vi "Anritsu VNA Read Trigger Mode.vi"(6 "Channel":i8=1 min=1 max=99 step=1, 7 "Anritsu VNA":T1, 8 "error in (no error)":errorcluster, 11 "VISA Resource Name":refnum<visa-resource-name>) -> (0 "error out":errorcluster, 2 "Trigger Mode":T2, 3 "dup VISA Resource Name":refnum<visa-resource-name>)   [LabVIEW 2011]
doc: "This VI for the HP8753B Network Analyzers reads the stimulus values. Except when performing log sweeps and freq list sweeps, this VI uses the start and stop values and the number of points to calcuate the stimulus values."
uses:
  TypeDefs/Anritsu VNA Trigger Mode.ctl
  TypeDefs/Anritsu VNA Instrument Info.ctl
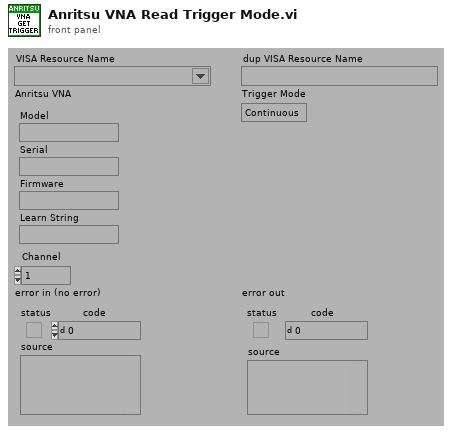
[diagram p1: front panel]
types:
  T1 = typedef "Anritsu VNA Instrument Info.ctl" = cluster{"Model":string, "Serial":string, "Firmware":string, "Learn String":string}
  T2 = typedef "Anritsu VNA Trigger Mode.ctl" = enum16{"Continuous", "Hold", "Single"}
  T3 = typedef "Anritsu VNA Model.ctl" = enum16{"Not Supported", "37XXXX", "MS20XXX", "MS462XX", "MS464XX"}
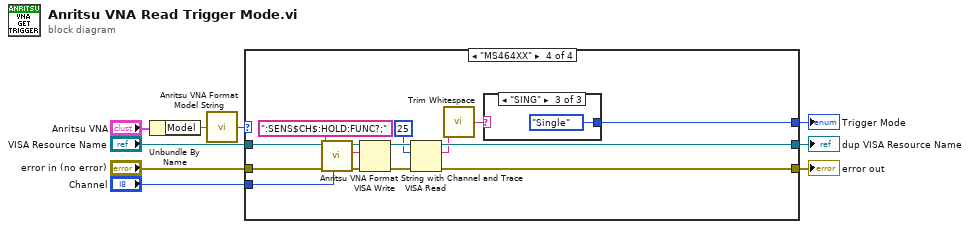
[diagram p0: block diagram]
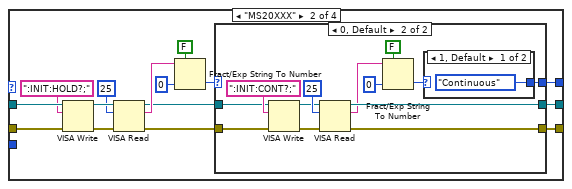
[diagram p3: hidden frame]
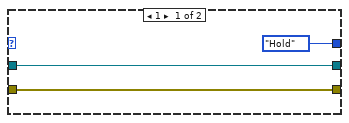
[diagram p4: hidden frame]
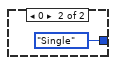
[diagram p5: hidden frame]
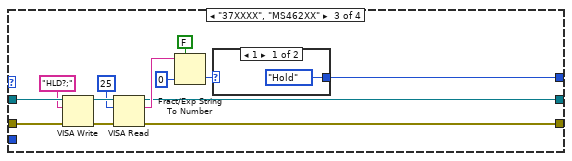
[diagram p6: hidden frame]
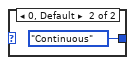
[diagram p7: hidden frame]
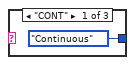
[diagram p8: hidden frame]
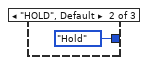
[diagram p9: hidden frame]
diagram:
  n1 = Unbundle By Name("Anritsu VNA") -> ("Model"=w3:string)
  n2 = call "Anritsu VNA Format Model String.vi"("Model"=w3) -> ("Model"=w2:T3)
  n3 = case shown="\"MS464XX\"" w2 {
    tunnel: "error in (no error)" -> [w10 w26 w57 w72]
    tunnel: [w10 w13 w46 w66] -> w8
    tunnel: "VISA Resource Name" -> [w11 w23 w54 w69]
    tunnel: [w11 w12 w45 w65] -> w6
    tunnel: [_ w17 w48 w67] -> w5
    tunnel: "Channel" -> [_ _ _ w62]
    frame "Not Supported" {
    }
    frame "MS20XXX" {
      n4 = VISA Write(VISA resource name=w23, write buffer=":INIT:HOLD?;", error in (no error)=w26) -> (VISA resource name out=w24:refnum<visa-resource-name>, error out=w25:errorcluster)  [unwired: 1 out]
      n5 = VISA Read(VISA resource name=w24, byte count=u32 25, error in (no error)=w25) -> (VISA resource name out=w15:refnum<visa-resource-name>, read buffer=w20:string, error out=w14:errorcluster)  [unwired: 1 out]
      n6 = Fract/Exp String To Number(use system decimal point (T)=FALSE, string=w20, default (0 dbl)=0 ("default (0 DBL)")) -> (number=w18:i32)  [unwired: 2 out]
      n7 = case shown="0, Default" w18 {
        tunnel: [Anritsu_VNA_Trigger_Mode."Hold" w42] -> w17
        tunnel: w15 -> [w28 w37]
        tunnel: w14 -> [w27 w36]
        tunnel: [w27 w35] -> w13
        tunnel: [w28 w34] -> w12
        frame 1 {
        }
        frame 0, Default {
          n8 = VISA Write(VISA resource name=w37, write buffer=":INIT:CONT?;", error in (no error)=w36) -> (VISA resource name out=w39:refnum<visa-resource-name>, error out=w38:errorcluster)  [unwired: 1 out]
          n9 = VISA Read(VISA resource name=w39, byte count=u32 25, error in (no error)=w38) -> (VISA resource name out=w34:refnum<visa-resource-name>, read buffer=w31:string, error out=w35:errorcluster)  [unwired: 1 out]
          n10 = Fract/Exp String To Number(use system decimal point (T)=FALSE, string=w31, default (0 dbl)=0 ("default (0 DBL)")) -> (number=w30:i32)  [unwired: 2 out]
          n11 = case shown="1, Default" w30 {
            tunnel: [Anritsu_VNA_Trigger_Mode."Continuous" Anritsu_VNA_Trigger_Mode."Single"] -> w42
            frame 1, Default {
            }
            frame 0 {
            }
          }
        }
      }
    }
    frame "37XXXX", "MS462XX" {
      n12 = VISA Write(VISA resource name=w54, write buffer="HLD?;", error in (no error)=w57) -> (VISA resource name out=w55:refnum<visa-resource-name>, error out=w56:errorcluster)  [unwired: 1 out]
      n13 = VISA Read(VISA resource name=w55, byte count=u32 25, error in (no error)=w56) -> (VISA resource name out=w45:refnum<visa-resource-name>, read buffer=w51:string, error out=w46:errorcluster)  [unwired: 1 out]
      n14 = Fract/Exp String To Number(use system decimal point (T)=FALSE, string=w51, default (0 dbl)=0 ("default (0 DBL)")) -> (number=w49:i32)  [unwired: 2 out]
      n15 = case shown="1" w49 {
        tunnel: [Anritsu_VNA_Trigger_Mode."Hold" Anritsu_VNA_Trigger_Mode."Continuous"] -> w48
        frame 1 {
        }
        frame 0, Default {
        }
      }
    }
    frame "MS464XX" {
      n16 = call "Anritsu VNA Format String with Channel and Trace.vi"("Channel"=w62, "String"=":SENS$CH$:HOLD:FUNC?;") -> ("String Out"=w63:string)  [unwired: 1 in, 6 out]
      n17 = VISA Write(VISA resource name=w69, write buffer=w63, error in (no error)=w72) -> (VISA resource name out=w70:refnum<visa-resource-name>, error out=w71:errorcluster)  [unwired: 1 out]
      n18 = VISA Read(VISA resource name=w70, byte count=u32 25, error in (no error)=w71) -> (VISA resource name out=w65:refnum<visa-resource-name>, read buffer=w61:string, error out=w66:errorcluster)  [unwired: 1 out]
      n19 = call <vilib>:"Trim Whitespace.vi"("string"=w61) -> ("trimmed string"=w60:string)  [unwired: 1 in]
      n20 = case shown="\"SING\"" w60 {
        tunnel: [Anritsu_VNA_Trigger_Mode."Continuous" Anritsu_VNA_Trigger_Mode."Hold" Anritsu_VNA_Trigger_Mode."Single"] -> w67
        frame "CONT" {
        }
        frame "HOLD", Default {
        }
        frame "SING" {
        }
      }
    }
  }
  "dup VISA Resource Name" <- w6
  "error out" <- w8
  "Trigger Mode" <- w5
